vi "Read ITX.vi"(8 "error in (no error)":errorcluster, 11 "Path":path) -> (0 "error out":errorcluster, 1 "Commands":string, 2 "Notes":string, 3 "Data (Dictionary)":T1[](array[typedef]))   [LabVIEW 2016, in "LV-Data.ITX.lvclass"]
uses:
  LV-Data.ITX.lvclass
  LV-Data/Typedefs/Dictionary--cluster.ctl
  LV-Data/LV-Data.lvclass
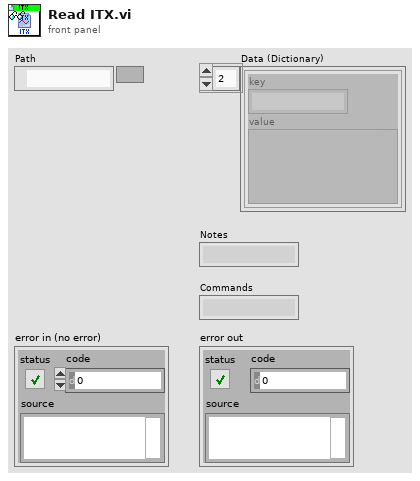
[diagram p1: front panel]
types:
  T1 = typedef "LV-Data.lvclass/Dictionary--cluster.ctl" = cluster{"key":string, "value":variant}
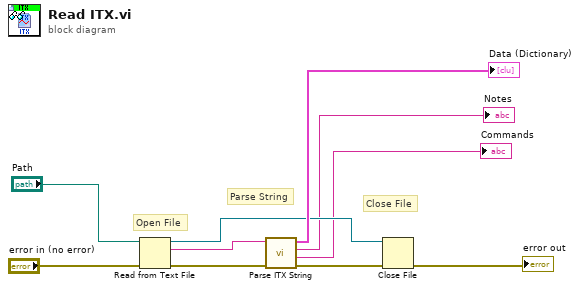
[diagram p0: block diagram]
diagram:
  # "Close File"
  # "Parse String"
  # "Open File"
  n1 = Read from Text File(file (use dialog)="Path", error in="error in (no error)") -> (refnum out=w5:refnum<file>, text=w1:string, error out=w7:errorcluster)  [unwired: 1 in, 2 out]
  n2 = call "Parse ITX String.vi"("error in (no error)"=w7, "ITX String"=w1) -> ("error out"=w8:errorcluster, "Commands"=→"Commands":string, "Notes"=→"Notes":string, "Array"=→"Data (Dictionary)":T1[])  [unwired: 6 in]
  n3 = Close File(refnum=w5, error in=w8) -> (error out=→"error out":errorcluster)  [unwired: 1 out]
